vi "TestDVRBuffer.vi"() -> ()   [LabVIEW 2017]
uses:
  <vilib>/addons/InsightCM/Devices/Shared/Common/DVRBuffer/DVRBuffer.lvlib
panel:
  out "Waveform Graph":waveform(sgl)[](graph)
  in  "buffer stop":ext
  in  "buffer start":ext
  out "found 2":bool
  out "waveforms":waveform(sgl)[](array[waveform])
  out "found":bool
  in  "location":ext
  out "write ptr monotonic":ext
  out "error out":errorcluster
  in  "stop":bool
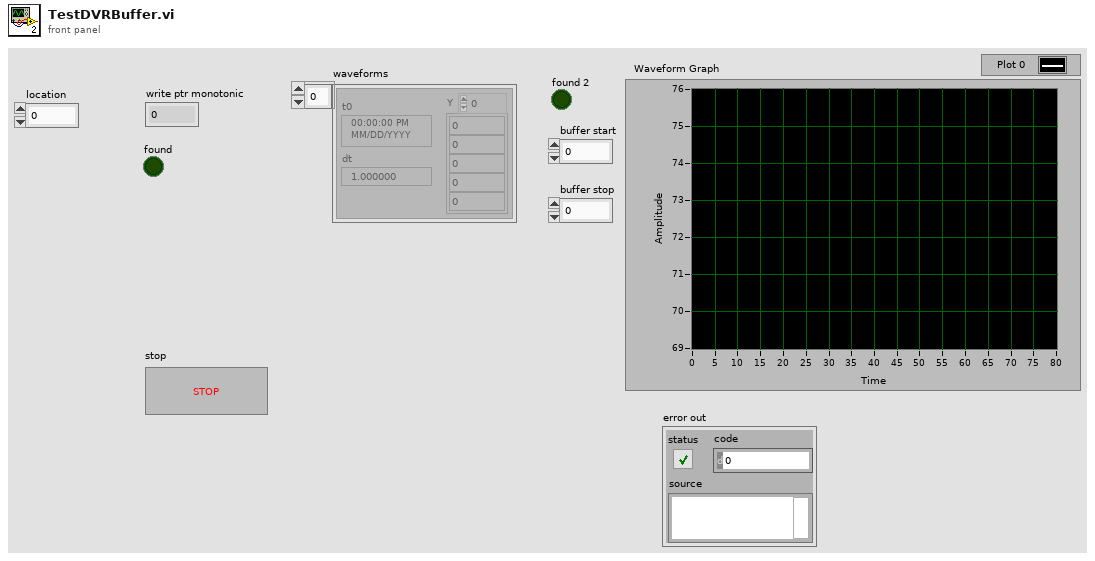
[diagram p1: front panel]
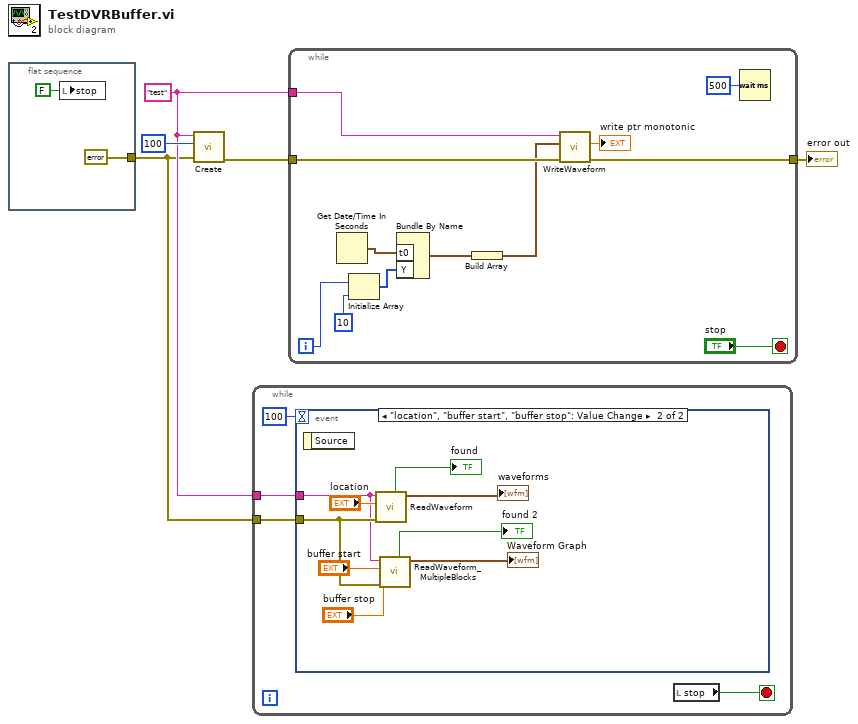
[diagram p0: block diagram]
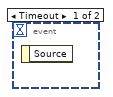
[diagram p2: hidden frame]
diagram:
  w2 = "test" ("name")
  n1 = flat-sequence {
    tunnel: [errorcluster {"status"=FALSE, "code"=0, "source"=""} ("error constant")] -> w1
    frame #0 {
      n2 = local write "stop"(FALSE ("stop")) -> ()
    }
  }
  n3 = call <vilib>:"Create.vi"("error in (no error)"=w1, "size"=100, "name"=w2) -> ("error out"=w5:errorcluster)  [unwired: 7 in, 1 out]
  n4 = while {
    tunnel: w2 -> [w10]
    tunnel: w1 -> [w8]
    stop <- w9 stop-if-true
    n5 = event shown="[1] \"location\", \"buffer start\", \"buffer stop\": Value Change" {
      selector: _ -> [_ _]
      dyn-events: _ -> [_ _]
      timeout: 100 -> [_ _]
      tunnel: w10 -> [_ w16]
      tunnel: w8 -> [_ w17]
      event Timeout {
        n6 = event-data() -> ()  [unwired: 1 in, 1 out]
      }
      event "location", "buffer start", "buffer stop": Value Change {
        n7 = event-data() -> ()  [unwired: 1 in, 1 out]
        n8 = call <vilib>:"ReadWaveform.vi"("error in (no error)"=w17, "buffer location"="location", "name"=w16) -> ("waveforms"=→"waveforms":waveform(sgl)[], "found"=→"found":bool)  [unwired: 6 in, 1 out]
        n9 = call <vilib>:"ReadWaveform_MultipleBlocks.vi"("error in (no error)"=w17, "buffer stop"="buffer stop", "buffer start"="buffer start", "name"=w16) -> ("waveforms"=→"Waveform Graph":waveform(sgl)[], "found"=→"found 2":bool)  [unwired: 5 in, 1 out]
      }
    }
    n10 = local read "stop"() -> (w9:bool)
  }
  n11 = while {
    tunnel: w5 -> [w32]
    tunnel: w2 -> [w31]
    tunnel: [w30] -> w3
    i -> [w23]
    stop <- "stop" stop-if-true
    n12 = Get Date/Time In Seconds() -> (seconds since 1Jan1904=w24:timestamp)
    n13 = Initialize Array(w23, 10 ("dimension size")) -> (w26:i32[])
    n14 = Bundle By Name("t0"=w24, "Y"=w26) -> (w22:waveform(i32))  [unwired: 1 in]
    n15 = Build Array(w22) -> (w21:waveform(i32)[])
    n16 = call <vilib>:"WriteWaveform.vi"("error in (no error)"=w32, "waveforms"=w21, "name"=w31) -> ("error out"=w30:errorcluster, "buffer location"=→"write ptr monotonic":ext)  [unwired: 7 in]
    n17 = Wait (ms)(milliseconds to wait=u32 500) -> ()  [unwired: 1 out]
  }
  "error out" <- w3
